vi "Set Value Test.vi"(8 "error in (no error)":errorcluster caption="entrée d'erreur (pas d'erreur)", 10 "Value Test":string, 11 "Class Camera  IV3-500CA - Start Program en entrée":refnum<class "Class Camera  IV3-500CA - Start Program.lvclass">) -> (0 "error out":errorcluster caption="sortie d'erreur", 3 "Class Camera  IV3-500CA - Start Program en sortie":refnum<class "Class Camera  IV3-500CA - Start Program.lvclass">)   [LabVIEW 2020, in "Library Instrument & Equipement.lvlib" / "Library Camera.lvlib" / "Class Camera  IV3-500CA - Start Program.lvclass"]
uses:
  Class Camera  IV3-500CA - Start Program.lvclass
  Class Camera  IV3-500CA - Start Program.lvclass/Class Camera  IV3-500CA - Start Program.ctl
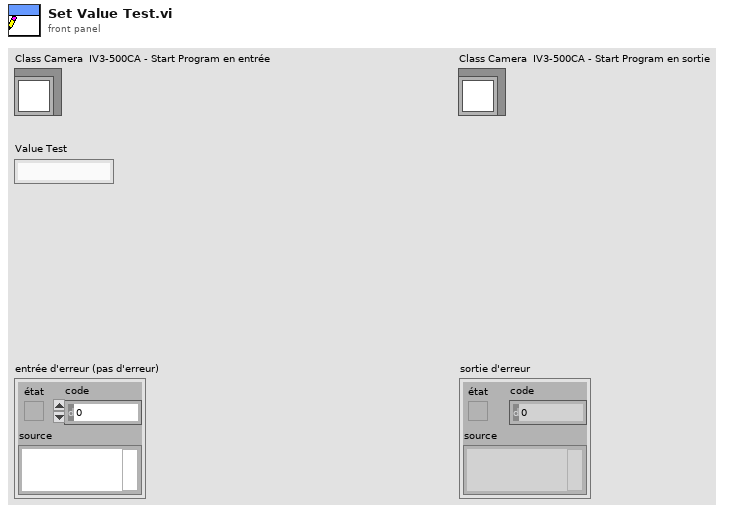
[diagram p1: front panel]
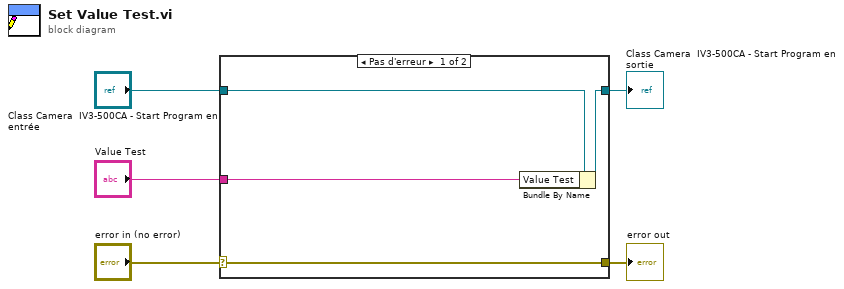
[diagram p0: block diagram]
diagram:
  n1 = case shown="Pas d'erreur" "error in (no error)" {
    selector: "error in (no error)" -> [w9 w10]
    tunnel: [w9 w10] -> w4
    tunnel: [w7 w11] -> w2
    tunnel: "Class Camera  IV3-500CA - Start Program en entrée" -> [w8 w11]
    tunnel: "Value Test" -> [w6 _]
    frame No Error {
      n2 = Bundle By Name(cluster=w8, "Value Test"=w6) -> (w7:refnum<class "Class Camera  IV3-500CA - Start Program.lvclass">)
    }
    frame Error {
    }
  }
  "error out" <- w4
  "Class Camera  IV3-500CA - Start Program en sortie" <- w2
